vi "Test con 568.vi"(1 "Equipo Nº":u8, 2 "Time Out":i32, 3 "Puerto:":u16, 5 "IP":string) -> (4 "Tx test color":u32, 6 "error out":errorcluster, 7 "RX tets color":u32, 8 "SEND":string, 9 "RETURN":string)   [LabVIEW 2010]
panel:
  out "data out":string
  out "comando":string
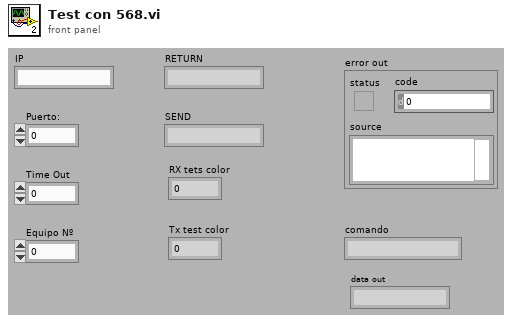
[diagram p1: front panel]
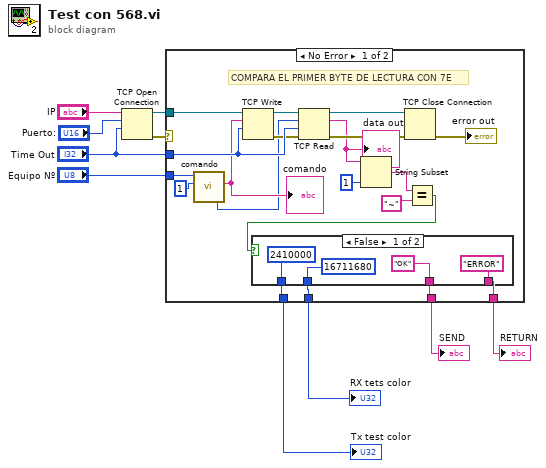
[diagram p0: block diagram]
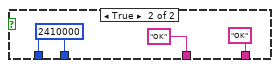
[diagram p2: hidden frame]
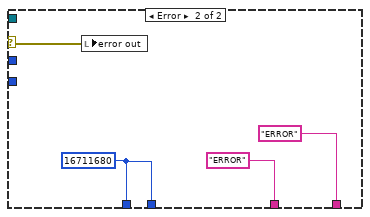
[diagram p3: hidden frame]
diagram:
  n1 = TCP Open Connection(address="IP", remote port or service name="Puerto:", timeout ms (60000)="Time Out") -> (connection ID=w4:refnum<k5>, error out=w9:errorcluster)  [unwired: 1 in, 1 out]
  n2 = case shown="No Error" w9 {
    selector: w9 -> [_ w38]
    tunnel: w4 -> [w30 _]
    tunnel: [w21 "ERROR" ("TEST?")] -> w7
    tunnel: [w26 w41] -> w5
    tunnel: "Time Out" -> [w28 _]
    tunnel: [w23 w41] -> w6
    tunnel: [w22 "ERROR" ("TEST?")] -> w8
    tunnel: "Equipo Nº" -> [w16 _]
    frame No Error {
      # "COMPARA EL PRIMER BYTE DE LECTURA CON 7E"
      n3 = call "comando.vi"("Comando:"=u8 1, "Equipo Nº"=w16) -> ("Bytes OUT"=w11:u16, "comando"=w13:string)  [unwired: 5 in]
      "comando" <- w13
      n4 = TCP Write(connection ID=w30, data in=w13, 9:w28) -> (connection ID out=w29:refnum<k5>, error out=w20:errorcluster)  [unwired: 1 in, 1 out]
      n5 = TCP Read(connection ID=w29, bytes to read=w11, error in (no error)=w20, 9:w28) -> (connection ID out=w25:refnum<k5>, data out=w12:string, error out=w19:errorcluster)  [unwired: 1 out]
      "data out" <- w12
      n6 = String Subset(string=w12, length (rest)=1 ("length (rest)")) -> (substring=w15:string)  [unwired: 1 in]
      n7 = TCP Close Connection(connection ID=w25, error in (no error)=w19) -> (error out=→"error out":errorcluster)  [unwired: 2 out]
      n8 = Equal?(x=w15, y="~" ("data in")) -> (x = y?=w24:bool)
      n9 = case shown="False" w24 {
        tunnel: ["OK" ("TEST?") "OK" ("TEST?")] -> w21
        tunnel: [u32 2410000 ("Text.Text Colors\n:Text Color") w36] -> w26
        tunnel: [u32 16711680 ("Text.Text Colors:Text Color") w36] -> w23
        tunnel: ["ERROR" ("TEST?") "OK" ("TEST?")] -> w22
        frame False {
        }
        frame True {
          w36 = u32 2410000 ("Text.Text Colors\n:Text Color")
        }
      }
    }
    frame Error {
      w41 = u32 16711680 ("Text.Text Colors:Text Color")
      n10 = local write "error out"(w38) -> ()
    }
  }
  "RETURN" <- w8
  "SEND" <- w7
  "RX tets color" <- w6
  "Tx test color" <- w5
